vi "SAVE in EXCEL.vi"() -> ()   [LabVIEW 2017]
uses:
  <vilib>/addons/_office/excel.llb/Excel Easy Table (str).vi
  <vilib>/Utility/NIReport.llb/NI_report.lvclass
  <vilib>/addons/_office/NI_ReportGenerationToolkit.lvlib
panel:
  in  "确定按钮 2":bool
  in  "数组":string[][](array[string])
  in  "确定按钮":bool
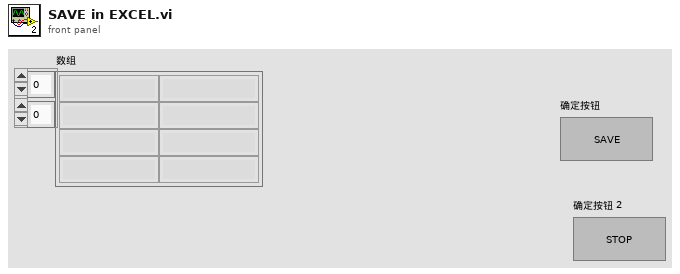
[diagram p1: front panel]
types:
  T1 = enum16{"maximized", "minimized", "normal", "no change"}
  T2 = enum16{"Standard Report", "HTML", "Word", "Excel"}
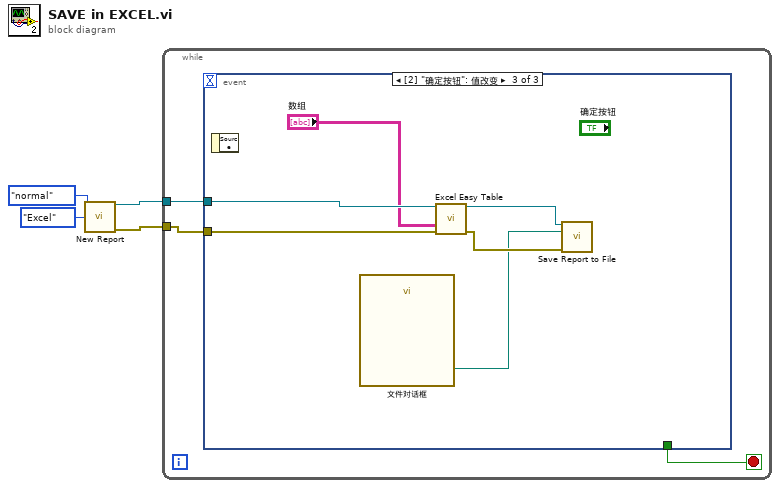
[diagram p0: block diagram]
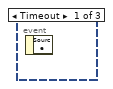
[diagram p2: hidden frame]
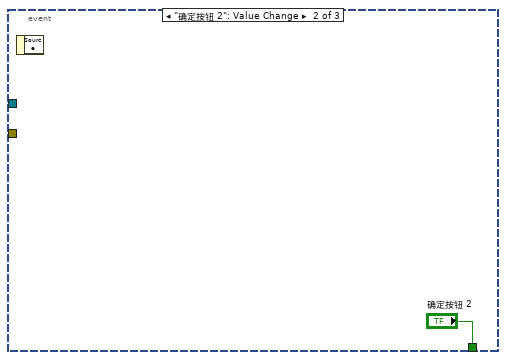
[diagram p3: hidden frame]
diagram:
  n1 = call <vilib>:"New Report.vi"("window state (normal)"=T1."normal", "report type"=T2."Excel") -> ("report out"=w4:refnum<class "NI_report.lvclass">, "error out"=w3:errorcluster)  [unwired: 12 in]
  n2 = while {
    tunnel: w4 -> [w6]
    tunnel: w3 -> [w5]
    stop <- w7 stop-if-true
    n3 = event shown="[2] \"确定按钮\": 值改变" {
      selector: _ -> [_ _ _]
      dyn-events: _ -> [_ _ _]
      timeout: _ -> [_ _ _]
      tunnel: [_ "确定按钮 2" _] -> w7
      tunnel: w6 -> [_ _ w14]
      tunnel: w5 -> [_ _ w13]
      event Timeout {
        n4 = event-data() -> ()  [unwired: 1 in, 1 out]
      }
      event "确定按钮 2": Value Change {
        n5 = event-data() -> ()  [unwired: 1 in, 1 out]
      }
      event "确定按钮": Value Change {
        n6 = event-data() -> ()  [unwired: 1 in, 1 out]
        n7 = call "文件对话框"() -> ("selected path"=w9:path)  [unwired: 12 in, 3 out]
        n8 = call-poly <vilib>:"Excel Easy Table.vi"("report in"=w14, "text data"="数组", "error in (no error)"=w13) -> ("report out"=w11:refnum<class "NI_report.lvclass">, "error out"=w10:errorcluster)  [unwired: 8 in, 3 out]
        n9 = call-dynamic "Save Report to File.vi"("report in"=w11, "report file path"=w9, "error in (no error)"=w10) -> ()  [unwired: 11 in, 2 out]
      }
    }
  }
